vi "Create Framework Configuration.vi"(11 "Plugins":T5(array[cluster])=[{"plugin class"="udp", "group configs"=[], "plugin timing"={"priority"=0, "decimation"=1, "offset"=0}, "settings"=[]}]) -> (3 "Framework Configuration":T6)   [LabVIEW 2017]
uses:
  Built/Engine/DSF.Engine.lvlibp/DSF Configuration API/1.0.0/Public/Controls/DSF Engine Framework Configuration.ctl
  Built/Engine/DSF.Engine.lvlibp/DSF Configuration API/1.0.0/Public/Controls/DSF Engine Plugin Configuration.ctl
  Built/Engine/DSF.Engine.lvlibp/DSF Configuration API/1.0.0/Public/Controls/DSF Timing Info.ctl
  Built/Engine/DSF.Engine.lvlibp/DSF Configuration API/1.0.0/Public/Controls/DSF Engine Transfer Group Configuration.ctl
  Built/Engine/DSF.Engine.lvlibp/DSF Configuration API/1.0.0/Public/Controls/DSF Direction.ctl
  Built/Engine/DSF.Engine.lvlibp/DSF Configuration API/1.0.0/Public/Controls/DSF Engine Transfer Configuration.ctl
  Built/Engine/DSF.Engine.lvlibp/DSF Configuration API/1.0.0/Public/Controls/DSF Byte Order.ctl
  Built/Engine/DSF.Engine.lvlibp/DSF Configuration API/1.0.0/Public/Controls/DSF Engine Channel Configuration.ctl
  Built/Engine/DSF.Engine.lvlibp/DSF Configuration API/1.0.0/Public/Controls/DSF Data Type.ctl
  Built/Engine/DSF.Engine.lvlibp/DSF Configuration API/1.0.0/Public/Controls/DSF Settings Info.ctl
  Source/DSF Configuration API/1.0.0/Public/Controls/DSF Direction.ctl
  Source/DSF Configuration API/1.0.0/Public/Controls/DSF Timing Info.ctl
  Built/Engine/DSF.Engine.lvlibp/DSF Configuration API/1.0.0/DSF Configuration API.lvlib
  Source/DSF Configuration API/1.0.0/DSF Configuration API.lvlib
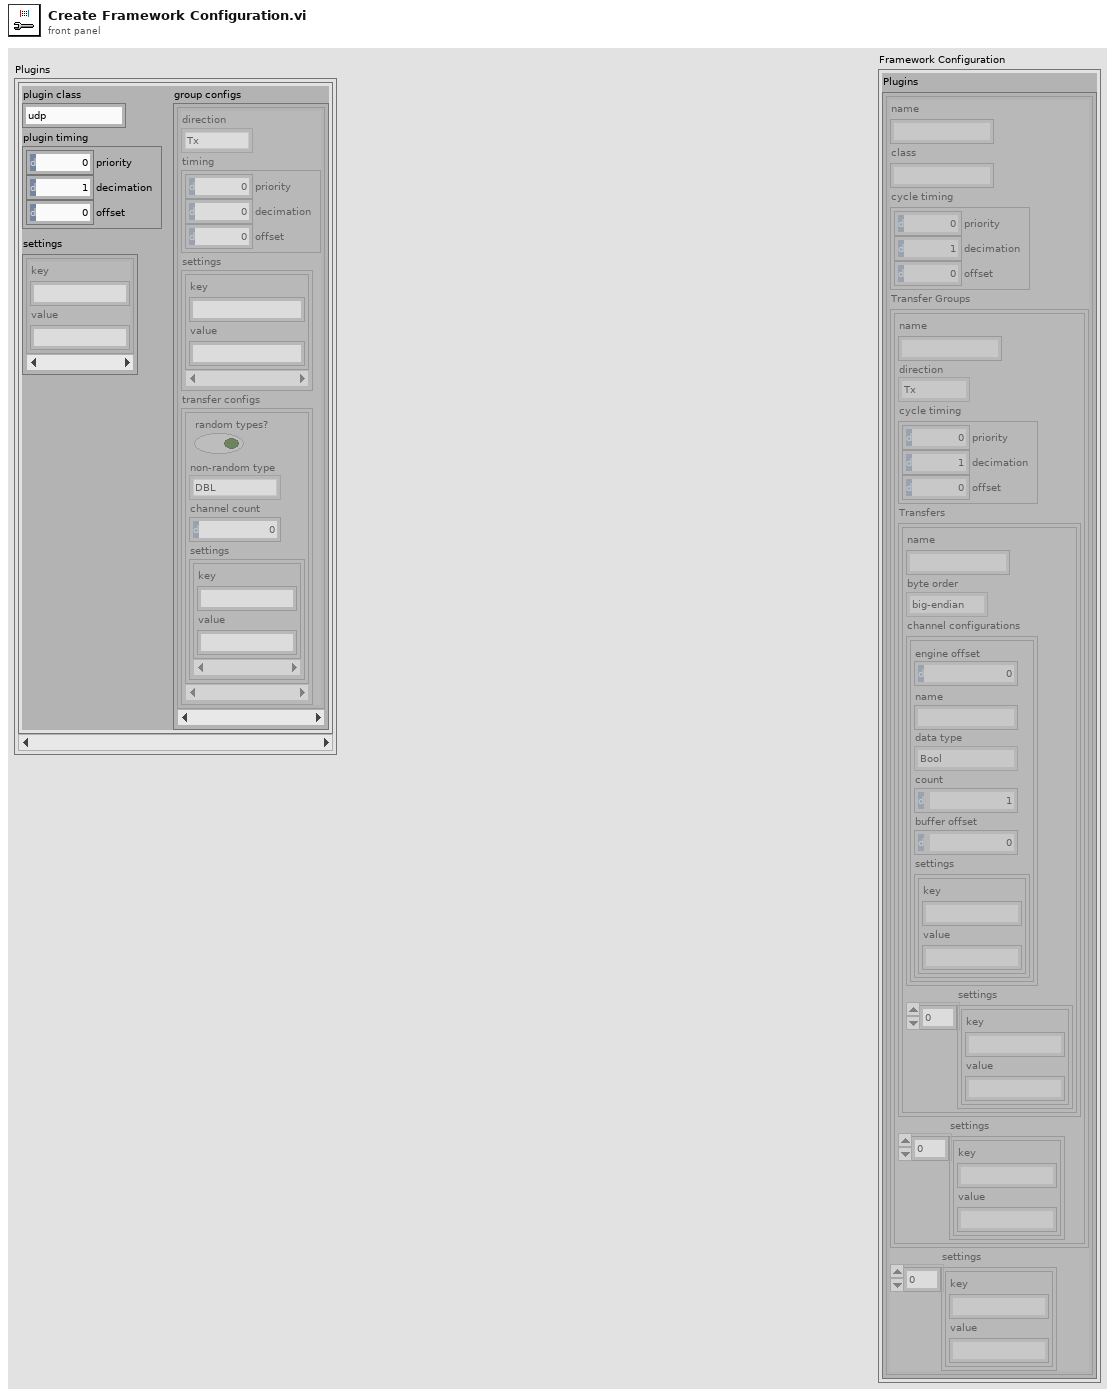
[diagram p1: front panel]
types:
  T1 = typedef "DSF Configuration API.lvlib/DSF Direction.ctl" = enum8{"Tx", "Rx"}
  T2 = typedef "DSF Configuration API.lvlib/DSF Timing Info.ctl" = cluster{"priority":u64, "decimation":u64, "offset":u64}
  T3 = typedef "DSF.Engine.lvlibp/DSF Configuration API.lvlib/DSF Settings Info.ctl" = cluster{"key":string, "value":string}[]
  T4 = typedef "DSF.Engine.lvlibp/DSF Configuration API.lvlib/DSF Data Type.ctl" = enum8{"Bool", "SGL", "DBL", "I8", "I16", "I32", "I64", "U8", "U16", "U32", "U64"}
  T5 = cluster{"plugin class":string, "group configs":cluster{"direction":T1, "timing":T2, "settings":T3, "transfer configs":cluster{"random types?":bool, "non-random type":T4, "channel count":i32, "settings":T3}[]}[], "plugin timing":T2, "settings":T3}[]
  T6 = typedef "DSF.Engine.lvlibp/DSF Configuration API.lvlib/DSF Engine Framework Configuration.ctl" = cluster{"Plugins":T7[]}
  T7 = typedef "DSF.Engine.lvlibp/DSF Configuration API.lvlib/DSF Engine Plugin Configuration.ctl" = cluster{"name":string, "class":string, "cycle timing":T8, "Transfer Groups":T9[], "settings":T3}
  T8 = typedef "DSF.Engine.lvlibp/DSF Configuration API.lvlib/DSF Timing Info.ctl" = cluster{"priority":u64, "decimation":u64, "offset":u64}
  T9 = typedef "DSF.Engine.lvlibp/DSF Configuration API.lvlib/DSF Engine Transfer Group Configuration.ctl" = cluster{"name":string, "direction":T10, "cycle timing":T8, "Transfers":T11[], "settings":T3}
  T10 = typedef "DSF.Engine.lvlibp/DSF Configuration API.lvlib/DSF Direction.ctl" = enum8{"Tx", "Rx"}
  T11 = typedef "DSF.Engine.lvlibp/DSF Configuration API.lvlib/DSF Engine Transfer Configuration.ctl" = cluster{"name":string, "byte order":T12, "channel configurations":T13[], "settings":T3}
  T12 = typedef "DSF.Engine.lvlibp/DSF Configuration API.lvlib/DSF Byte Order.ctl" = enum8{"big-endian", "little-endian"}
  T13 = typedef "DSF.Engine.lvlibp/DSF Configuration API.lvlib/DSF Engine Channel Configuration.ctl" = cluster{"engine offset":u64, "name":string, "data type":T4, "count":u64, "buffer offset":u64, "settings":T3}
  T14 = cluster{"direction":T1, "timing":T2, "settings":T3, "transfer configs":cluster{"random types?":bool, "non-random type":T4, "channel count":i32, "settings":T3}[]}[]
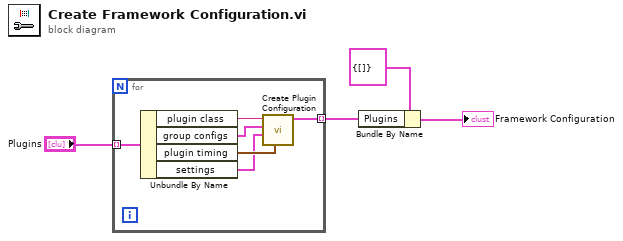
[diagram p0: block diagram]
diagram:
  n1 = for {
    tunnel: [w10] -> w1 mode=indexing
    tunnel: "Plugins" -> [w9] mode=indexing
    n2 = Unbundle By Name(w9) -> ("plugin class"=w8:string, "group configs"=w6:T14, "plugin timing"=w7:T2, "settings"=w5:T3)
    n3 = call "Create Plugin Configuration.vi"("plugin timing"=w7, "settings"=w5, "group configs"=w6, "plugin class"=w8) -> ("Plugin Configuration"=w10:T7)  [unwired: 7 in]
  }
  n4 = Bundle By Name(cluster=T6 {"Plugins"=[]} ("Framework Configuration"), "Plugins"=w1) -> (→"Framework Configuration":T6)
